vi "SetDisplayText.vi"(8 "Error In":errorcluster, 9 "Text (32 Characters)":string, 10 "Window":u8=1 min=1 max=2 step=1, 11 "Keithley 6482 In":refnum<visa-resource-name>) -> (0 "Error Out":errorcluster, 3 "Keithley 6482 Out":refnum<visa-resource-name>)   [LabVIEW 2014, in "Keithley-6482-Visa.lvlib"]
uses:
  Keithley-6482-Visa.lvlib
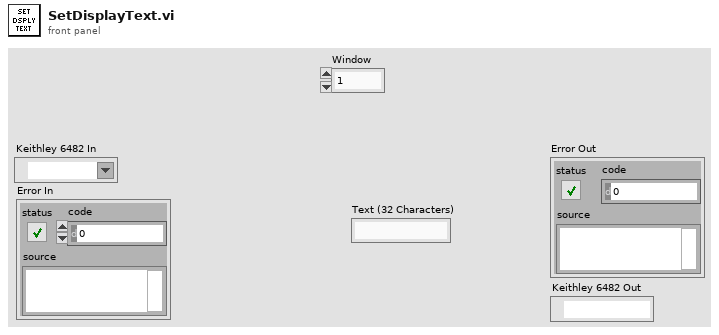
[diagram p1: front panel]
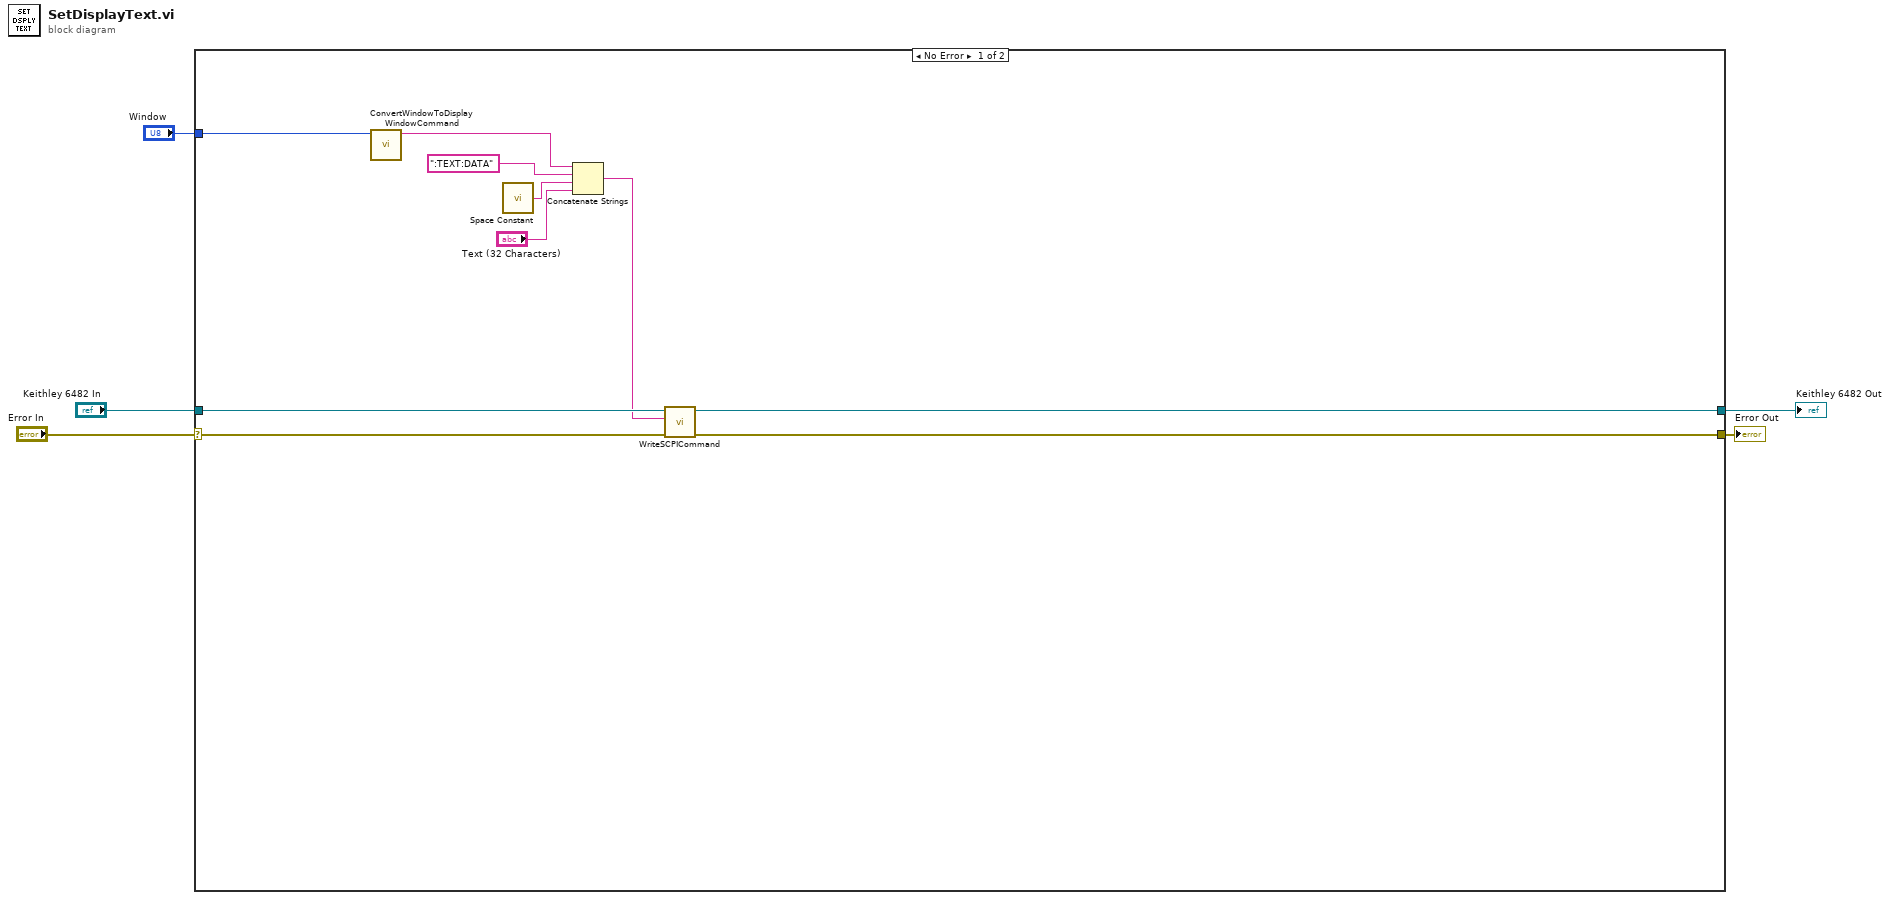
[diagram p0: block diagram]
diagram:
  n1 = case shown="No Error" "Error In" {
    selector: "Error In" -> [w11 w16]
    tunnel: "Keithley 6482 In" -> [w14 w17]
    tunnel: [w12 w16] -> w3
    tunnel: [w13 w17] -> w2
    tunnel: "Window" -> [w7 _]
    frame No Error {
      n2 = call "ConvertWindowToDisplayWindowCommand.vi"("Window"=w7) -> ("Display Window Command"=w6:string)  [unwired: 10 in]
      n3 = call <vilib>:"Space Constant.vi"() -> ("String"=w15:string)
      n4 = Concatenate Strings(w6, ":TEXT:DATA", w15, "Text (32 Characters)") -> (w10:string)
      n5 = call "WriteSCPICommand.vi"("Error In"=w11, "SCPI Command"=w10, "Keithley 6482 In"=w14) -> ("Error Out"=w12:errorcluster, "Keithley 6482 Out"=w13:refnum<visa-resource-name>)  [unwired: 7 in]
    }
    frame Error {
    }
  }
  "Error Out" <- w3
  "Keithley 6482 Out" <- w2
